vi "Clear and Flush Table.vi"(8 "error in":errorcluster, 11 "Table in":refnum<vi>) -> (0 "error out":errorcluster)   [LabVIEW 2025, in "Automotive Ethernet Bus Monitor UI.lvlib"]
doc: "Clear the Referenced Table and Flush the Table Buffer."
uses:
  Automotive Ethernet Bus Monitor UI.lvlib
  <vilib>/Utility/miscctls.llb/LVRowAndColumnTypeDef.ctl
  Flush Table.vi
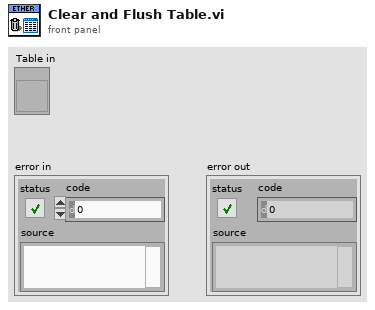
[diagram p1: front panel]
types:
  T1 = typedef "LVRowAndColumnTypeDef.ctl" = cluster{"Row":i32, "Column":i32}
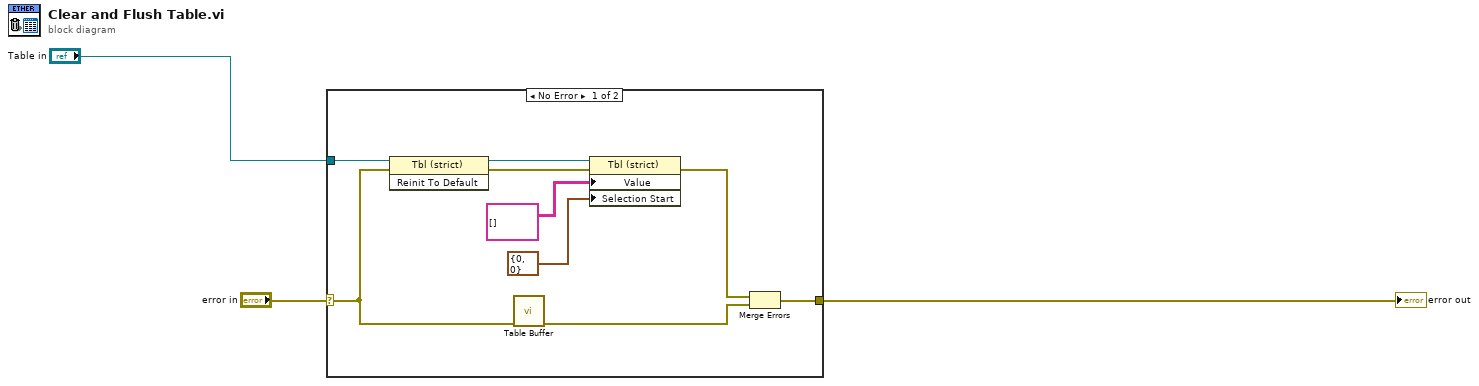
[diagram p0: block diagram]
diagram:
  n1 = case shown="No Error" "error in" {
    selector: "error in" -> [w4 w13]
    tunnel: "Table in" -> [w10 _]
    tunnel: [w6 w13] -> w2
    frame No Error {
      n2 = invoke class="Tbl (strict)" method="Reinit To Default"(reference=w10, error in=w4) -> (reference out=w11:refnum<vi>, error out=w12:errorcluster)  [unwired: 1 in, 1 out]
      n3 = call-poly "Table Buffer.vi"("error in"=w4) -> ("error out"=w5:errorcluster)  [unwired: 10 in]
      n4 = property class="Tbl (strict)"(reference=w11, error in=w12, "Value"=string[][] [], "Selection Start"=T1 {"Row"=0, "Column"=0}) -> (error out=w7:errorcluster)  [unwired: 1 out]
      n5 = Merge Errors(w7, w5) -> (w6:errorcluster)
    }
    frame Error {
    }
  }
  "error out" <- w2
